vi "Node - PXImc Write.vi"(8 "error in (no error)":errorcluster, 10 "Writer Data In":u8[](array[numeric]), 11 "Node Data In":T1) -> (0 "error out":errorcluster, 3 "Node Data Out":T1)   [LabVIEW 2016, in "PXImc Router.lvlib"]
uses:
  PXImc Router.lvlib
  Controls/Node/Node - Config.ctl
  <vilib>/NI Veristand/VeriStand Data/Byte Buffer/Byte Buffer.lvclass
  Controls/Node/Node - PXImc Parameters.ctl
  Controls/Node/Node - Writer Data.ctl
  Controls/Node/Node - Ch Properties.ctl
  Controls/Data Type.ctl
  Controls/Node/Node - Readers Data.ctl
  Controls/Node/Node - Reader Data.ctl
  <vilib>/pximc/Acquire Write Region (U8).vi
  <vilib>/pximc/nipximc.lvlib
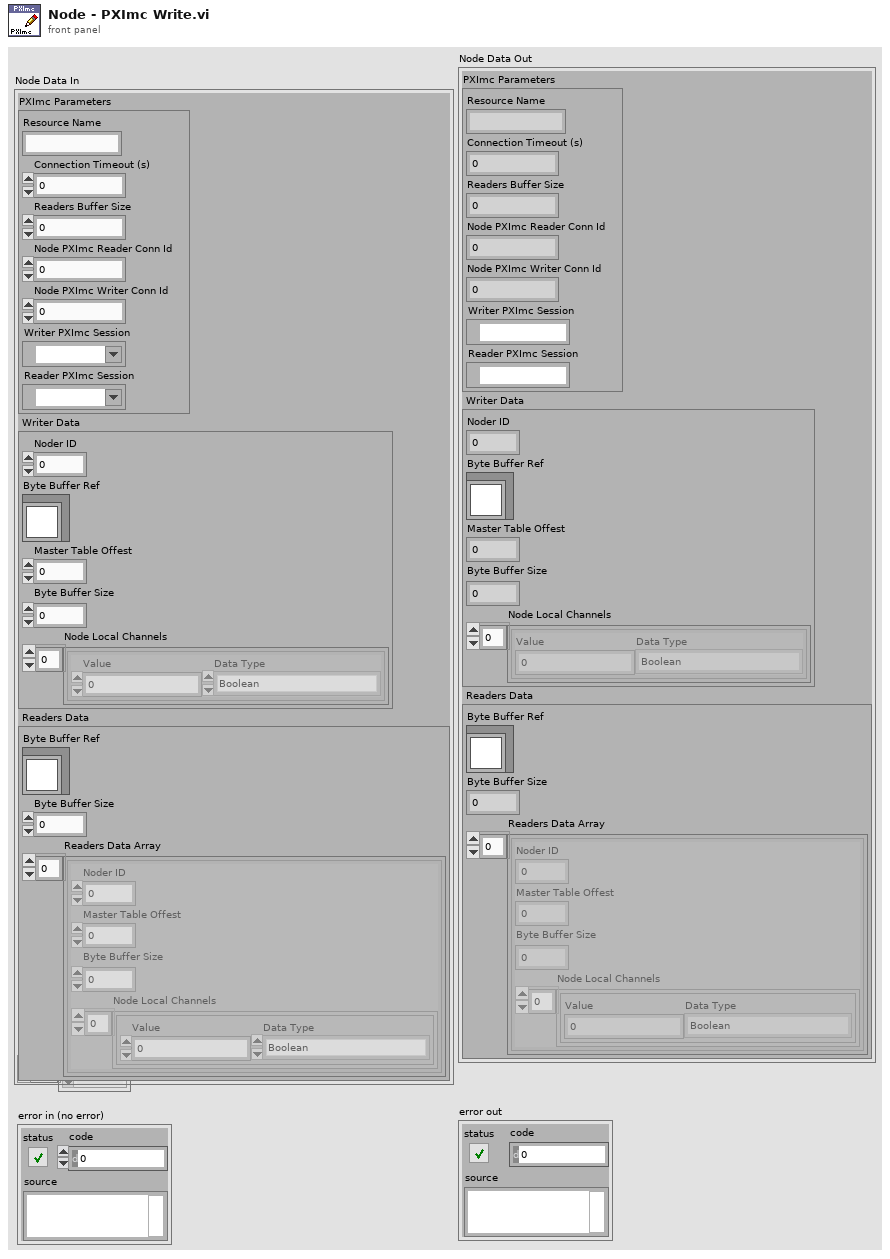
[diagram p1: front panel]
types:
  T1 = typedef "PXImc Router.lvlib/Node - Config.ctl" = cluster{"PXImc Parameters":T2, "Writer Data":T3, "Readers Data":T6}
  T2 = typedef "PXImc Router.lvlib/Node - PXImc Parameters.ctl" = cluster{"Resource Name":string, "Connection Timeout (s)":dbl, "Readers Buffer Size":u64, "Node PXImc Reader Conn Id":u16, "Node PXImc Writer Conn Id":u16, "Writer PXImc Session":refnum<k21>, "Reader PXImc Session":refnum<k21>}
  T3 = typedef "PXImc Router.lvlib/Node - Writer Data.ctl" = cluster{"Noder ID":u32, "Byte Buffer Ref":refnum<class "Byte Buffer.lvclass">, "Master Table Offest":u32, "Byte Buffer Size":u32, "Node Local Channels":T4[]}
  T4 = typedef "PXImc Router.lvlib/Node - Ch Properties.ctl" = cluster{"Value":dbl, "Data Type":T5}
  T5 = typedef "PXImc Router.lvlib/Data Type.ctl" = enum16{"Boolean", "SGL", "DBL", "I8", "I16", "I32", "I64", "U8", "U16", "U32", "U64"}
  T6 = typedef "PXImc Router.lvlib/Node - Readers Data.ctl" = cluster{"Byte Buffer Ref":refnum<class "Byte Buffer.lvclass">, "Byte Buffer Size":u64, "Readers Data Array":T7[]}
  T7 = typedef "PXImc Router.lvlib/Node - Reader Data.ctl" = cluster{"Noder ID":u32, "Master Table Offest":u32, "Byte Buffer Size":u64, "Node Local Channels":T4[]}
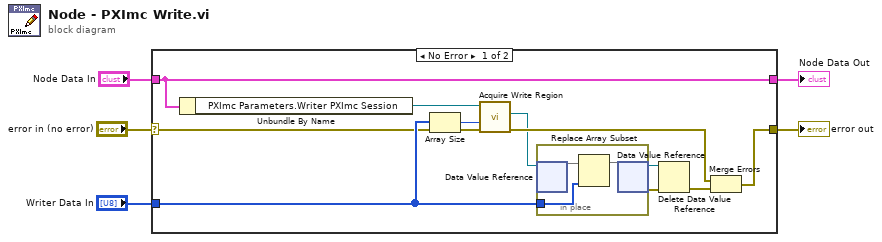
[diagram p0: block diagram]
diagram:
  n1 = case shown="No Error" "error in (no error)" {
    selector: "error in (no error)" -> [w7 w21]
    tunnel: "Writer Data In" -> [w16 _]
    tunnel: [w9 w21] -> w4
    tunnel: "Node Data In" -> [w6 w20]
    tunnel: [w6 w20] -> w1
    frame No Error {
      n2 = Unbundle By Name(w6) -> ("PXImc Parameters.Writer PXImc Session"=w8:refnum<k21>)
      n3 = Array Size(array=w16) -> (size(s)=w15:i32)
      n4 = call-poly <vilib>:"Acquire Write Region.vi"("error in (no error)"=w7, "number of elements"=w15, "session in"=w8) -> ("error out"=w14:errorcluster, "write region reference"=w13:refnum<data-value>)  [unwired: 5 in, 2 out]
      n5 = in-place {
        in-place-border: w16 -> [w17]
        n6 = in-place-dvr #1(w13) -> (w19:u8[])  [unwired: 1 out]
        n7 = Replace Array Subset(array=w19, new element=w17) -> (w18:u8[])  [unwired: 1 in]
        n8 = in-place-dvr #1(w18) -> (w12:refnum<data-value>, w10:errorcluster)
      }
      n9 = Delete Data Value Reference(data value reference=w12, error in=w10) -> (error out=w11:errorcluster)  [unwired: 1 out]
      n10 = Merge Errors(w14, w11) -> (w9:errorcluster)
    }
    frame Error {
    }
  }
  "error out" <- w4
  "Node Data Out" <- w1
